vi "Reference_Test.vi"() -> ()   [LabVIEW 2017, in "WordManipulationTests.lvlib"]
uses:
  WordManipulationTests.lvlib
  Utilities/ReferenceMoveParameters.ctl
  Utilities/WordManipulationLibrary.lvlib
panel:
  out "Failed?":bool
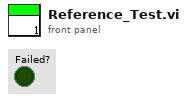
[diagram p1: front panel]
types:
  T1 = typedef "WordManipulationLibrary.lvlib/ReferenceMoveParameters.ctl" = cluster{"Reference Move Mode":i32, "Start Search Forward":bool, "Stop on FWD Edge":bool, "Approach Forward":bool, "Velocity":dbl, "Acceleration":dbl}
  T2 = cluster{"Reference Move Mode":bool, "Start Search Forward":bool, "Stop on FWD Edge":bool, "Approach Forward":bool, "Velocity":bool, "Acceleration":bool}
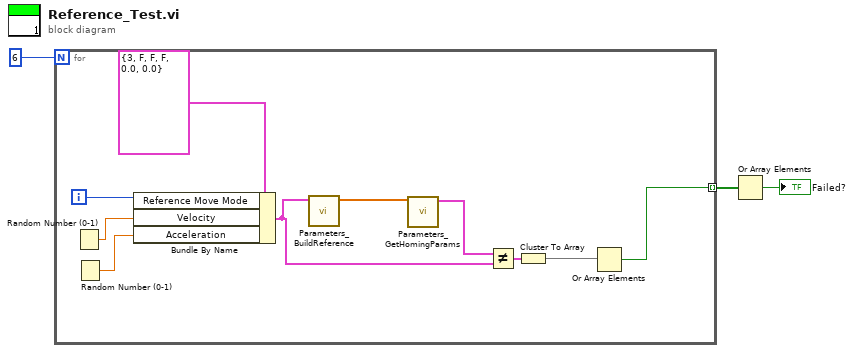
[diagram p0: block diagram]
diagram:
  n1 = for {
    N: 6 -> [_]
    tunnel: [w5] -> w1 mode=indexing
    i -> [w12]
    n2 = Random Number (0-1)() -> (number: 0 to 1=w11:dbl)
    n3 = Random Number (0-1)() -> (number: 0 to 1=w10:dbl)
    n4 = Bundle By Name(cluster=T1 {"Reference Move Mode"=3, "Start Search Forward"=FALSE, "Stop on FWD Edge"=FALSE, "Approach Forward"=FALSE, "Velocity"=0.0, "Acceleration"=0.0} ("Reference Move Parameters"), "Reference Move Mode"=w12, "Velocity"=w11, "Acceleration"=w10) -> (w8:T1)
    n5 = call "Parameters_BuildReference.vi"("Reference Move Parameters"=w8) -> ("Parameters"=w4:dbl[])  [unwired: 10 in]
    n6 = call "Parameters_GetHomingParams.vi"("Parameters"=w4) -> ("Reference Move Parameters"=w9:T1)  [unwired: 9 in, 1 out]
    n7 = Not Equal?(x=w9, y=w8) -> (x != y?=w7:T2)
    n8 = Cluster To Array(cluster=w7) -> (array=w6:bool[])
    n9 = Or Array Elements(Boolean array=w6) -> (logical OR=w5:bool)
  }
  n10 = Or Array Elements(Boolean array=w1) -> (logical OR=→"Failed?":bool)
